vi "Demo - Hardware in the Loop Application.vi"() -> ()   [LabVIEW 2017]
doc: "This application demonstrates the basic application of the hardware in the loop mode.\n\n-Initialises and configures the device\n-Uploads data the arbitrary waveform generator\n-Runs a shot\n-Downloads the data and displays it\n-Changes the data\n-Repeats the process"
uses:
  Communications/Typedefs/Data Size--Enum.ctl
  Communications/Communications Library.lvlib
  GUI/Consoles/Communications Console Library.lvlib
panel:
  in  "Analog In Data Size":T1
  in  "Display Console":bool
  in  "INI File Path":path caption="INI File Path (Blank for Defaults)"
  out "Ready":bool
  out "error out":errorcluster
  out "Number of Shots Run":i32
  in  "stop":bool
  in  "Channel":i32
  in  "Speed":dbl=0.5 format="%#_13g"
  out "Data Received":bool
  out "Shot Completed":bool
  in  "Samples to Read":i32=80000
  in  "Length of AO Data (Samples)":i32=32768
  out "Analog Input Plot":i32[][](graph)
  out "Analog Output Plot":i16[][](graph)
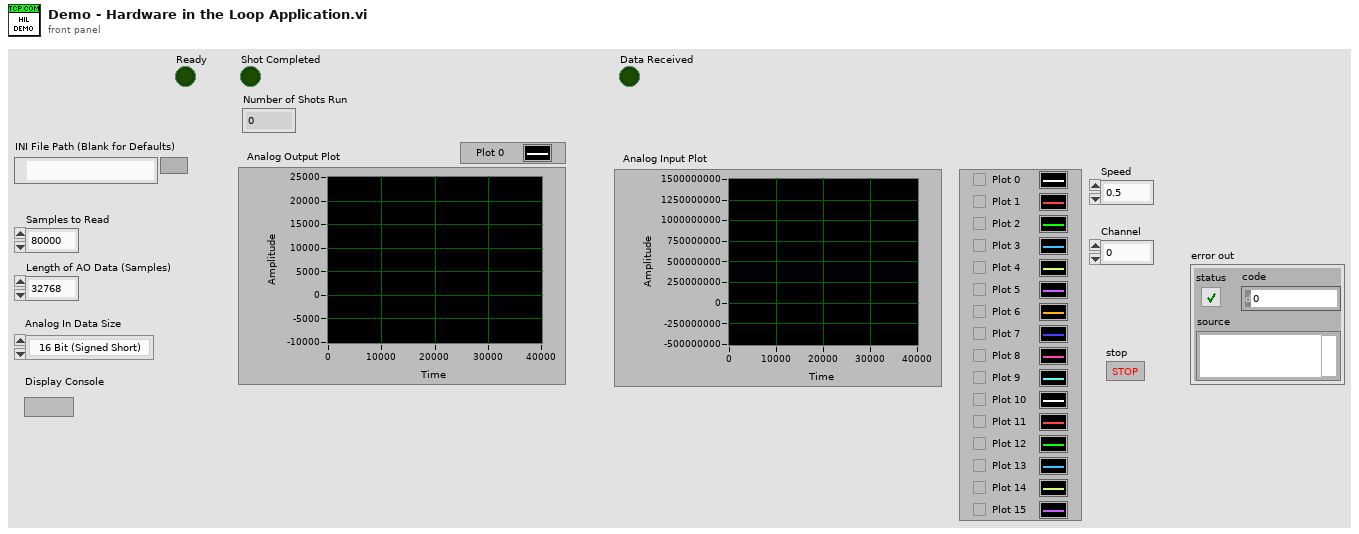
[diagram p1: front panel]
types:
  T1 = typedef "Communications Library.lvlib/Data Size--Enum.ctl" = enum16{"16 Bit (Signed Short)", "32 Bit (Signed Long)"}
  T2 = typedef "Communications Library.lvlib/DTACQ Module Carrier Configuration--Cluster.ctl" = cluster{"Name":string, "IP":string, "Control Port":i32, "Timeout (ms)":i32, "Continuous Capture Port (Multiplexed)":i32, "Start HIL Shot Port":i32, "AWG Upload Port (Multiplexed)":i32, "Download Captured Data Port (Multiplexed)":i32, "Module Slots":i32, "Module Configurations":T3[]}
  T3 = typedef "Communications Library.lvlib/DTACQ Module Configuration--Cluster.ctl" = cluster{"Name":string, "Position":string, "Module Type":T4, "Control Port":i32, "Timeout (ms)":i32, "Channels":i32}
  T4 = typedef "Communications Library.lvlib/DTACQ Device Type--Enum.ctl" = enum16{"Carrier", "Analog In Module", "Analog Out Module", "Generic Module"}
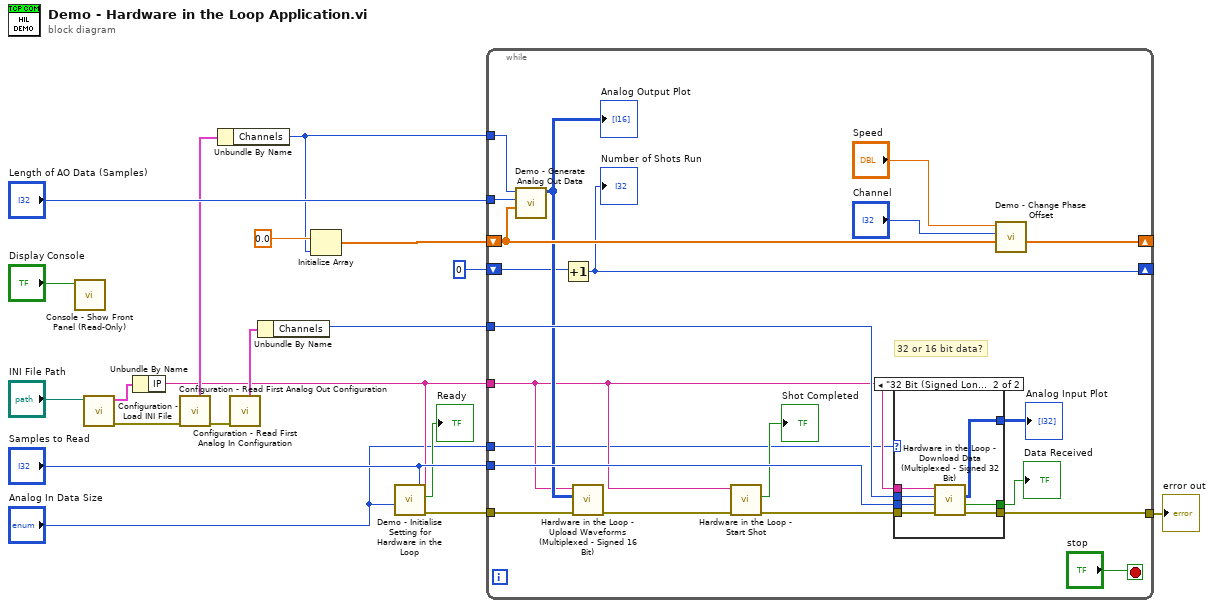
[diagram p0: block diagram]
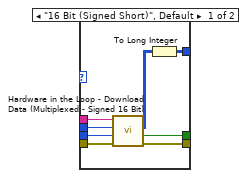
[diagram p2: hidden frame]
diagram:
  n1 = call "Console - Show Front Panel (Read-Only).vi"("Display Console"="Display Console") -> ()  [unwired: 11 in]
  n2 = call "Configuration - Load INI File.vi"("configuration file path"="INI File Path") -> ("error out"=w12:errorcluster, "Carrier Configuration Out"=w6:T2)  [unwired: 9 in]
  n3 = Unbundle By Name(w6) -> ("IP"=w5:string)
  n4 = call "Configuration - Read First Analog Out Configuration.vi"("error in"=w12) -> ("error out"=w11:errorcluster, "AO - Module Configuration"=w10:T3)  [unwired: 6 in, 3 out]
  n5 = Unbundle By Name(w10) -> ("Channels"=w9:i32)
  n6 = call "Configuration - Read First Analog In Configuration.vi"("error in"=w11) -> ("AI - Module Configuration"=w8:T3)  [unwired: 6 in, 4 out]
  n7 = Unbundle By Name(w8) -> ("Channels"=w7:i32)
  n8 = Initialize Array(0.0, w9) -> (w17:dbl[])
  n9 = call "Demo - Initialise Setting for Hardware in the Loop.vi"("Analog In Data Size"="Analog In Data Size", "Samples to Read"="Samples to Read", "Address"=w5) -> ("error out"=w3:errorcluster, "Ready"=→"Ready":bool)  [unwired: 7 in]
  n10 = while {
    tunnel: w5 -> [w29]
    tunnel: w7 -> [w40]
    tunnel: "Samples to Read" -> [w39]
    tunnel: "Length of AO Data (Samples)" -> [w37]
    tunnel: w9 -> [w38]
    shift-right: [w33] -> _
    shift-left: w17 -> [w34]
    tunnel: [w35] -> w18
    shift-right: [w30] -> _
    shift-left: 0 -> [w31]
    tunnel: w3 -> [w28]
    tunnel: "Analog In Data Size" -> [w21]
    stop <- "stop" stop-if-true
    # "32 or 16 bit data?"
    n11 = call "Demo - Generate Analog Out Data.vi"("Phase Offset (Radians)"=w34, "Number of Samples"=w37, "Number of AO Channels"=w38) -> ("Sine Wave"=w32:i16[][])  [unwired: 8 in]
    "Analog Output Plot" <- w32
    n12 = Increment(x=w31) -> (x+1=w30:i32)
    "Number of Shots Run" <- w30
    n13 = call "Hardware in the Loop - Upload Waveforms (Multiplexed - Signed 16 Bit).vi"("error in"=w28, "Multichannel Waveform"=w32, "Address"=w29) -> ("error out"=w25:errorcluster)  [unwired: 8 in]
    n14 = call "Hardware in the Loop - Start Shot.vi"("error in"=w25, "Address"=w29) -> ("error out"=w24:errorcluster, "Shot Completed"=→"Shot Completed":bool)  [unwired: 8 in]
    n15 = case shown="\"32 Bit (Signed Long)\"" w21 {
      tunnel: w40 -> [w48 w50]
      tunnel: w39 -> [w47 w49]
      tunnel: [w46 w54] -> w35
      tunnel: w29 -> [w45 w51]
      tunnel: w24 -> [w44 w55]
      tunnel: [w43 w53] -> w22
      tunnel: [w41 w52] -> w20
      frame "16 Bit (Signed Short)", Default {
        n16 = call "Hardware in the Loop - Download Data (Multiplexed - Signed 16 Bit).vi"("error in"=w44, "Number of Samples"=w47, "Number of Channels"=w48, "Address"=w45) -> ("error out"=w46:errorcluster, "Data Received"=w43:bool, "Data"=w42:i16[][])  [unwired: 5 in]
        n17 = To Long Integer(number=w42) -> (32bit integer=w41:i32[][])
      }
      frame "32 Bit (Signed Long)" {
        n18 = call "Hardware in the Loop - Download Data (Multiplexed - Signed 32 Bit).vi"("error in"=w55, "Number of Samples"=w49, "Number of Channels"=w50, "Address"=w51) -> ("error out"=w54:errorcluster, "Data Received"=w53:bool, "Data"=w52:i32[][])  [unwired: 5 in]
      }
    }
    "Analog Input Plot" <- w20
    "Data Received" <- w22
    n19 = call "Demo - Change Phase Offset.vi"("Phase Offset (Radians) in"=w34, "Channel"="Channel", "x"="Speed") -> ("Phase Offset (Radians) out"=w33:dbl[])  [unwired: 8 in]
  }
  "error out" <- w18
